vi "Report File Data Log Sample.vi"(8 "error in (no error)":errorcluster, 10 "Data Row":dbl[](array[numeric]), 11 "Report File in":refnum<class "Report File.lvclass">) -> (0 "error out":errorcluster, 3 "Report File out":refnum<class "Report File.lvclass">)   [LabVIEW 2018, in "Report File.lvclass"]
uses:
  Report File.lvclass
  Report File.lvclass/Report File.ctl
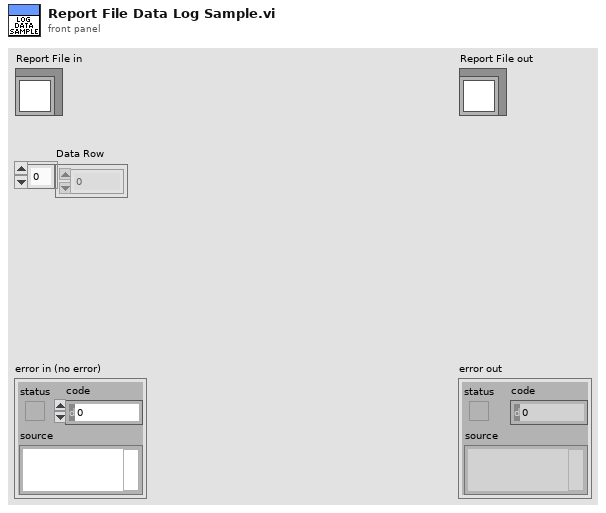
[diagram p1: front panel]
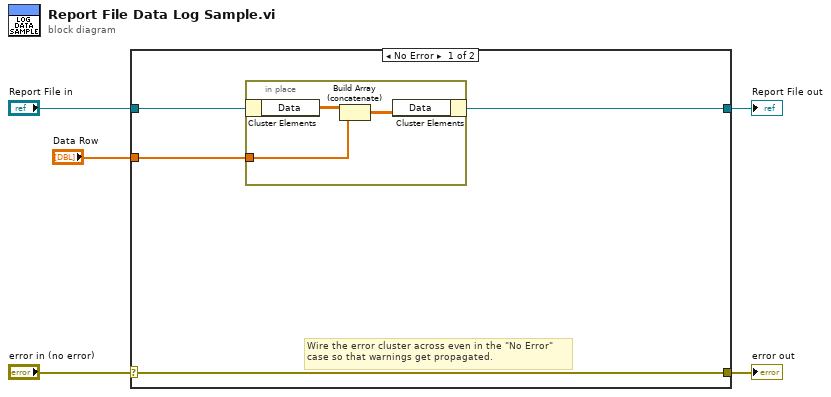
[diagram p0: block diagram]
diagram:
  n1 = case shown="No Error" "error in (no error)" {
    selector: "error in (no error)" -> [w9 w14]
    tunnel: [w9 w14] -> w4
    tunnel: [w7 w13] -> w2
    tunnel: "Report File in" -> [w8 w13]
    tunnel: "Data Row" -> [w6 _]
    frame No Error {
      # "Wire the error cluster across even in the \"No Error\"\ncase so that warnings get propagated."
      n2 = in-place {
        in-place-border: w6 -> [w11]
        n3 = in-place-cluster #1(w8) -> ("Data"=w12:dbl[][])
        n4 = Build Array (concatenate)(w12, w11) -> (w10:dbl[][])
        n5 = in-place-cluster #1("Data"=w10) -> (w7:refnum<class "Report File.lvclass">)
      }
    }
    frame Error {
    }
  }
  "error out" <- w4
  "Report File out" <- w2
